vi "Error Dialog.vi"(8 "error in (no error)":errorcluster, 11 "Instrument in":refnum<class "Instrument.lvclass">) -> (0 "error out":errorcluster, 2 "States to Execute":string, 3 "Instrument out":refnum<class "Instrument.lvclass">)   [LabVIEW 2016, in "Instrument.lvclass"]
uses:
  Instrument.lvclass
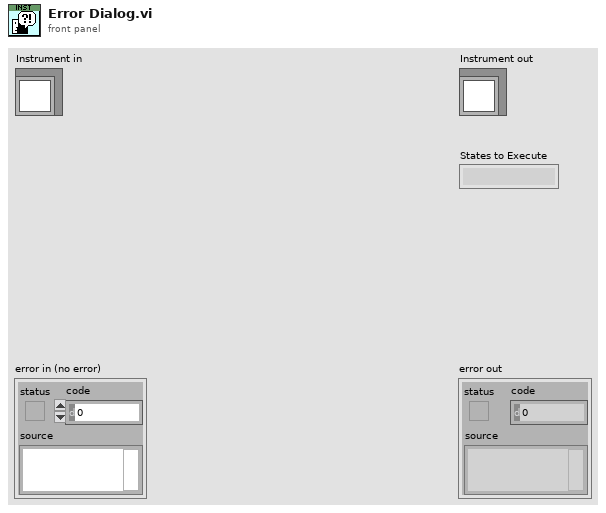
[diagram p1: front panel]
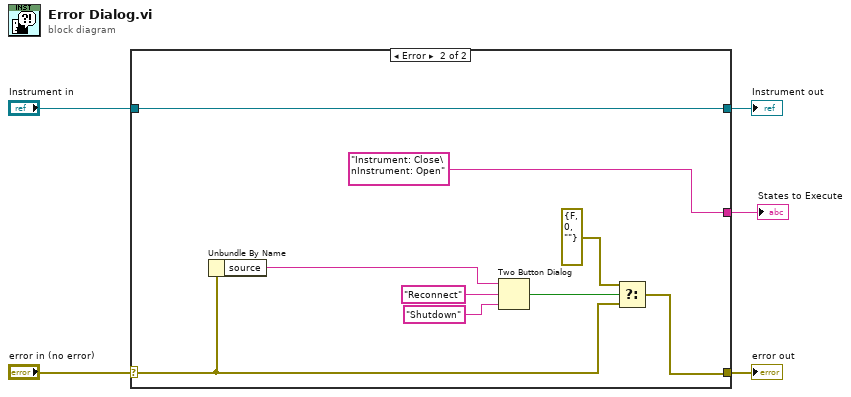
[diagram p0: block diagram]
diagram:
  n1 = case shown="Error" "error in (no error)" {
    selector: "error in (no error)" -> [w6 w9]
    tunnel: [w6 w14] -> w4
    tunnel: [w7 w16] -> w2
    tunnel: "Instrument in" -> [w7 w16]
    tunnel: [_ "Instrument: Close\nInstrument: Open" ("States to Execute")] -> w1
    frame No Error {
      # "Wire the error cluster across even in the \"No Error\"\ncase so that warnings get propagated."
    }
    frame Error {
      n2 = Unbundle By Name(w9) -> ("source"=w8:string)
      n3 = Two Button Dialog(message=w8, 1:"Shutdown" ("F button name (\"Cancel\")"), 2:"Reconnect" ("T button name (\"OK\")")) -> (T button?=w13:bool)
      n4 = Select(t=errorcluster {"status"=FALSE, "code"=0, "source"=""} ("error constant"), s=w13, f=w9) -> (s? t:f=w14:errorcluster)
    }
  }
  "error out" <- w4
  "Instrument out" <- w2
  "States to Execute" <- w1
